vi "Point Distances.vi"(11 "Points":cluster{"X":sgl, "Y":sgl}[](array[cluster]) {"Y" format="%.2f"; "X" format="%.2f"}) -> (3 "Distances":sgl[](array[numeric]) format="%.4f")   [LabVIEW 2025]
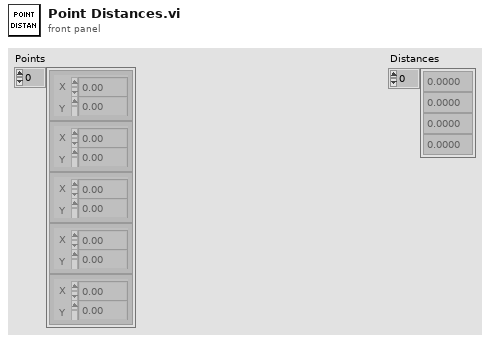
[diagram p1: front panel]
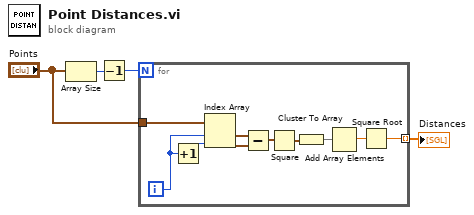
[diagram p0: block diagram]
diagram:
  n1 = Array Size(array="Points") -> (size(s)=w4:i32)
  n2 = Decrement(x=w4) -> (x-1=w3:i32)
  n3 = for {
    N: w3 -> [_]
    tunnel: "Points" -> [w14]
    tunnel: [w5] -> w1 mode=indexing
    i -> [w12]
    n4 = Increment(x=w12) -> (x+1=w13:i32)
    n5 = Index Array(array=w14, index #1=w12, index #2=w13) -> (element #1=w11:cluster{"X":sgl, "Y":sgl}, element #2=w10:cluster{"X":sgl, "Y":sgl})
    n6 = Subtract(x=w11, y=w10) -> (x-y=w9:cluster{"X":sgl, "Y":sgl})
    n7 = Square(x=w9) -> (x^2=w8:cluster{"X":sgl, "Y":sgl})
    n8 = Cluster To Array(cluster=w8) -> (array=w7:sgl[])
    n9 = Add Array Elements(numeric array=w7) -> (sum=w6:sgl)
    n10 = Square Root(x=w6) -> (sqrt(x)=w5:sgl)
  }
  "Distances" <- w1
